vi "Icon_Build 2D Image from Image Cluster.vi"(8 "Error":errorcluster, 11 "Color256":T2={"image type"=0, "image depth"=8, "image"=[210, 210, 210, 210, 210, 210, 210, 210, 210, 210, 210, 210, 210, 210, 210, 210, 210, 210, 210, 210, 210, 210, 210, 210, 210, 210, 210, 210, 210, 210, 210, 210, 210, 210, 210, 210, 210, 210, 5, 5, 5, 210, 210, 5, 5, 210, 210, 210, 5, 5, 5, 210, 210, 5, 210, 210, 210, 5, 210, 210, 210, 210, 210, 210, 210, 210, 210, 210, 210, 210, 210, 5, 210, 210, 5, 210, 210, 5, 210, 5, 210, 210, 210, 5, 210, 5, 5, 210, 210, 5, 210, 210, 210, 210, 210, 210, 210, 210, 210, 210, 210, 210, 210, 5, 210, 210, 5, 210, 210, 210, 210, 5, 210, 210, 210, 5, 210, 5, 210, 5, 210, 5, 210, 210, 210, 210, 210, 210, 210, 210, 210, 210, 210, 210, 210, 5, 210, 210, 5, 210, 210, 5, 210, 5, 210, 210, 210, 5, 210, 5, 210, 210, 5, 5, 210, 210, 210, 210, 210, 210, 210, 210, 210, 210, 210, 210, 5, 5, 5, 210, 210, 5, 5, 210, 210, 210, 5, 5, 5, 210, 210, 5, 210, 210, 210, 5, 210, 210, 210, 210, 210, 210, 210, 210, 210, 210, 210, 210, 210, 210, 210, 210, 210, 210, 210, 210, 210, 210, 210, 210, 210, 210, 210, 210, 210, 210, 210, 210, 210, 210, 210, 210, 210, 210, 210, 5, 5, 5, 5, 5, 5, 5, 5, 5, 5, 5, 5, 5, 5, 5, 5, 5, 5, 5, 5, 5, 5, 5, 5, 5, 5, 5, 5, 5, 5, 210, 210, 5, 5, 5, 5, 5, 5, 5, 5, 5, 5, 5, 5, 5, 5, 5, 5, 5, 5, 5, 5, 5, 5, 5, 5, 5, 5, 5, 5, 5, 5, 210, 210, 5, 5, 5, 5, 5, 5, 5, 5, 5, 5, 5, 5, 5, 5, 5, 5, 5, 5, 5, 5, 5, 5, 5, 5, 5, 5, 5, 5, 5, 5, 210, 210, 5, 5, 210, 210, 5, 5, 210, 210, 210, 5, 5, 210, 210, 210, 210, 5, 5, 210, 210, 5, 5, 210, 210, 210, 5, 210, 210, 210, 210, 5, 210, 210, 5, 210, 5, 5, 210, 5, 210, 5, 5, 210, 5, 210, 5, 5, 5, 5, 210, 5, 5, 210, 5, 5, 210, 5, 5, 210, 5, 5, 5, 5, 210, 210, 5, 210, 5, 5, 5, 5, 210, 210, 210, 5, 5, 210, 210, 210, 5, 5, 210, 210, 210, 210, 5, 5, 210, 5, 5, 210, 210, 210, 5, 5, 210, 210, 5, 210, 5, 5, 210, 5, 210, 5, 5, 210, 5, 210, 5, 5, 5, 5, 210, 5, 5, 210, 5, 5, 210, 5, 5, 210, 5, 5, 5, 5, 210, 210, 5, 5, 210, 210, 5, 5, 210, 5, 5, 210, 5, 210, 210, 210, 210, 5, 210, 5, 5, 210, 5, 5, 210, 5, 5, 210, 210, 210, 210, 5, 210, 210, 5, 5, 5, 5, 5, 5, 5, 5, 5, 5, 5, 5, 5, 5, 5, 5, 5, 5, 5, 5, 5, 5, 5, 5, 5, 5, 5, 5, 5, 5, 210, 210, 5, 5, 5, 5, 5, 5, 5, 5, 5, 5, 5, 5, 5, 5, 5, 5, 5, 5, 5, 5, 5, 5, 5, 5, 5, 5, 5, 5, 5, 5, 210, 210, 5, 5, 5, 5, 5, 5, 5, 5, 5, 5, 5, 210, 210, 210, 5, 5, 210, 210, 210, 5, 5, 5, 5, 5, 5, 5, 5, 5, 5, 5, 210, 210, 5, 5, 5, 5, 5, 5, 5, 5, 5, 5, 5, 5, 5, 5, 210, 5, 210, 5, 5, 210, 5, 5, 5, 5, 5, 5, 5, 5, 5, 5, 210, 210, 5, 5, 5, 5, 5, 5, 5, 5, 5, 5, 5, 5, 210, 210, 5, 5, 210, 5, 5, 210, 5, 5, 5, 5, 5, 5, 5, 5, 5, 5, 210, 210, 5, 5, 5, 5, 5, 5, 5, 5, 5, 5, 5, 210, 5, 5, 5, 5, 210, 5, 5, 210, 5, 5, 5, 5, 5, 5, 5, 5, 5, 5, 210, 210, 5, 5, 5, 5, 5, 5, 5, 5, 5, 5, 5, 210, 210, 210, 210, 5, 210, 210, 210, 5, 5, 5, 5, 5, 5, 5, 5, 5, 5, 5, 210, 210, 5, 5, 5, 5, 5, 5, 5, 5, 5, 5, 5, 5, 5, 5, 5, 5, 5, 5, 5, 5, 5, 5, 5, 5, 5, 5, 5, 5, 5, 5, 210, 210, 5, 5, 5, 5, 5, 5, 5, 5, 5, 5, 5, 5, 5, 5, 5, 5, 5, 5, 5, 5, 5, 5, 5, 5, 5, 5, 5, 5, 5, 5, 210, 210, 5, 5, 5, 5, 210, 210, 5, 5, 210, 210, 210, 5, 5, 210, 210, 210, 5, 5, 5, 210, 210, 5, 5, 210, 5, 5, 5, 210, 5, 5, 210, 210, 5, 5, 5, 210, 5, 5, 210, 5, 210, 5, 5, 210, 5, 210, 5, 5, 210, 5, 210, 5, 5, 210, 5, 5, 210, 5, 210, 5, 5, 5, 210, 210, 5, 5, 5, 210, 210, 210, 210, 5, 210, 210, 210, 5, 5, 210, 210, 210, 5, 5, 210, 210, 210, 210, 5, 5, 5, 210, 5, 5, 5, 5, 210, 210, 5, 5, 5, 210, 5, 5, 210, 5, 210, 5, 5, 210, 5, 210, 5, 5, 210, 5, 210, 5, 5, 210, 5, 5, 5, 210, 5, 5, 5, 5, 210, 210, 5, 5, 5, 210, 5, 5, 210, 5, 210, 5, 5, 210, 5, 210, 5, 5, 210, 5, 210, 5, 5, 210, 5, 5, 5, 210, 5, 5, 5, 5, 210, 210, 5, 5, 5, 5, 5, 5, 5, 5, 5, 5, 5, 5, 5, 5, 5, 5, 5, 5, 5, 5, 5, 5, 5, 5, 5, 5, 5, 5, 5, 5, 210, 210, 5, 5, 5, 5, 5, 5, 5, 5, 5, 5, 5, 5, 5, 5, 5, 5, 5, 5, 5, 5, 5, 5, 5, 5, 5, 5, 5, 5, 5, 5, 210, 210, 210, 210, 210, 210, 210, 210, 210, 210, 210, 210, 210, 210, 210, 210, 210, 210, 210, 210, 210, 210, 210, 210, 210, 210, 210, 210, 210, 210, 210, 210, 210], "mask"=[255, 255, 255, 255, 255, 255, 255, 255, 255, 255, 255, 255, 255, 255, 255, 255, 255, 255, 255, 255, 255, 255, 255, 255, 255, 255, 255, 255, 255, 255, 255, 255, 255, 255, 255, 255, 255, 255, 255, 255, 255, 255, 255, 255, 255, 255, 255, 255, 255, 255, 255, 255, 255, 255, 255, 255, 255, 255, 255, 255, 255, 255, 255, 255, 255, 255, 255, 255, 255, 255, 255, 255, 255, 255, 255, 255, 255, 255, 255, 255, 255, 255, 255, 255, 255, 255, 255, 255, 255, 255, 255, 255, 255, 255, 255, 255, 255, 255, 255, 255, 255, 255, 255, 255, 255, 255, 255, 255, 255, 255, 255, 255, 255, 255, 255, 255, 255, 255, 255, 255, 255, 255, 255, 255, 255, 255, 255, 255], "colors"=[16777215, 16777164, 16777113, 16777062, 16777011, 16776960, 16764159, 16764108, 16764057, 16764006, 16763955, 16763904, 16751103, 16751052, 16751001, 16750950, 16750899, 16750848, 16738047, 16737996, 16737945, 16737894, 16737843, 16737792, 16724991, 16724940, 16724889, 16724838, 16724787, 16724736, 16711935, 16711884, 16711833, 16711782, 16711731, 16711680, 13434879, 13434828, 13434777, 13434726, 13434675, 13434624, 13421823, 13421772, 13421721, 13421670, 13421619, 13421568, 13408767, 13408716, 13408665, 13408614, 13408563, 13408512, 13395711, 13395660, 13395609, 13395558, 13395507, 13395456, 13382655, 13382604, 13382553, 13382502, 13382451, 13382400, 13369599, 13369548, 13369497, 13369446, 13369395, 13369344, 10092543, 10092492, 10092441, 10092390, 10092339, 10092288, 10079487, 10079436, 10079385, 10079334, 10079283, 10079232, 10066431, 10066380, 10066329, 10066278, 10066227, 10066176, 10053375, 10053324, 10053273, 10053222, 10053171, 10053120, 10040319, 10040268, 10040217, 10040166, 10040115, 10040064, 10027263, 10027212, 10027161, 10027110, 10027059, 10027008, 6750207, 6750156, 6750105, 6750054, 6750003, 6749952, 6737151, 6737100, 6737049, 6736998, 6736947, 6736896, 6724095, 6724044, 6723993, 6723942, 6723891, 6723840, 6711039, 6710988, 6710937, 6710886, 6710835, 6710784, 6697983, 6697932, 6697881, 6697830, 6697779, 6697728, 6684927, 6684876, 6684825, 6684774, 6684723, 6684672, 3407871, 3407820, 3407769, 3407718, 3407667, 3407616, 3394815, 3394764, 3394713, 3394662, 3394611, 3394560, 3381759, 3381708, 3381657, 3381606, 3381555, 3381504, 3368703, 3368652, 3368601, 3368550, 3368499, 3368448, 3355647, 3355596, 3355545, 3355494, 3355443, 3355392, 3342591, 3342540, 3342489, 3342438, 3342387, 3342336, 65535, 65484, 65433, 65382, 65331, 65280, 52479, 52428, 52377, 52326, 52275, 52224, 39423, 39372, 39321, 39270, 39219, 39168, 26367, 26316, 26265, 26214, 26163, 26112, 13311, 13260, 13209, 13158, 13107, 13056, 255, 204, 153, 102, 51, 15597568, 14483456, 12255232, 11141120, 8912896, 7798784, 5570560, 4456448, 2228224, 1114112, 60928, 56576, 47872, 43520, 34816, 30464, 21760, 17408, 8704, 4352, 238, 221, 187, 170, 136, 119, 85, 68, 34, 17, 15658734, 14540253, 12303291, 11184810, 8947848, 7829367, 5592405, 4473924, 2236962, 1118481, 0], "Rectangle"={"left"=0, "top"=0, "right"=32, "bottom"=32}}) -> (0 "Error Out":errorcluster, 3 "2D Image Out":T1)   [LabVIEW 2009]
uses:
  Controls/Cluster/Cluster_Image Data.ctl
  Controls/Cluster/CLuster_Selectoin Box.ctl
  Controls/Array/Color Box Array_2D Icon Viewer.ctl
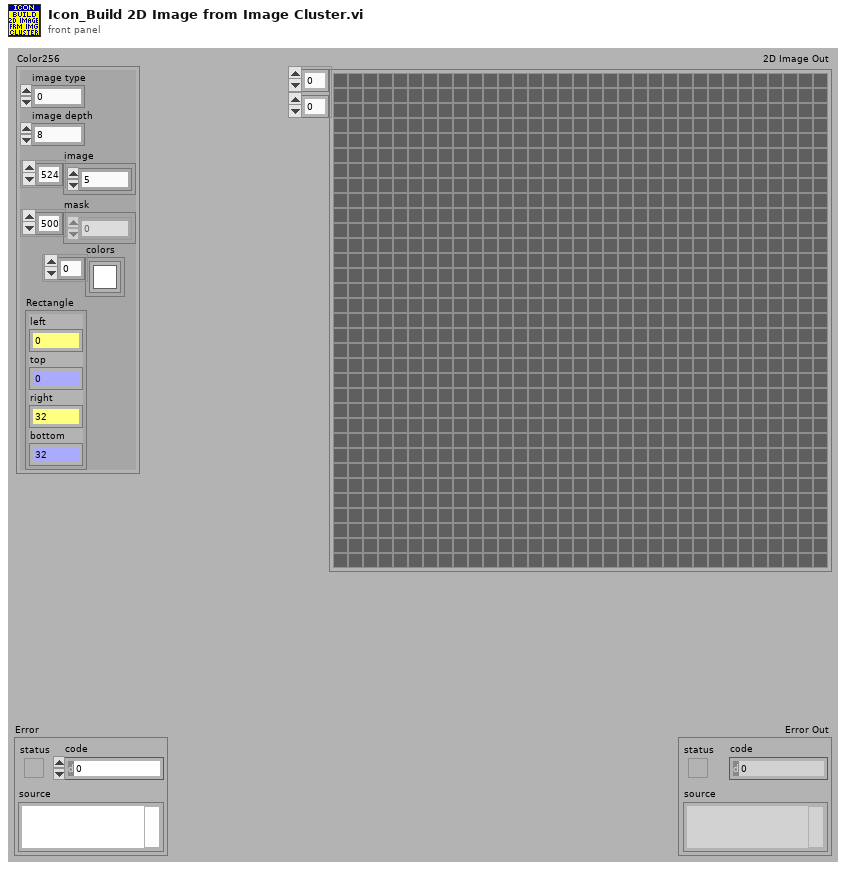
[diagram p1: front panel]
types:
  T1 = typedef "Color Box Array_2D Icon Viewer.ctl" = u32[][]
  T2 = typedef "Cluster_Image Data.ctl" = cluster{"image type":i32, "image depth":i32, "image":u8[], "mask":u8[], "colors":u32[], "Rectangle":T3}
  T3 = typedef "CLuster_Selectoin Box.ctl" = cluster{"left":i16, "top":i16, "right":i16, "bottom":i16}
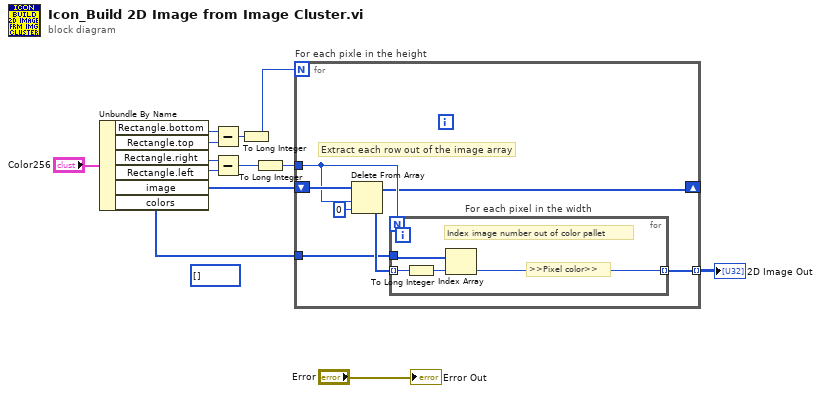
[diagram p0: block diagram]
diagram:
  (unwired) u32[] [] ("colors")
  n1 = Unbundle By Name("Color256") -> ("Rectangle.bottom"=w6:i16, "Rectangle.top"=w5:i16, "Rectangle.right"=w13:i16, "Rectangle.left"=w12:i16, "image"=w9:u8[], "colors"=w8:u32[])
  n2 = Subtract(x=w6, y=w5) -> (x-y=w11:i16)
  n3 = Subtract(x=w13, y=w12) -> (x-y=w10:i16)
  n4 = To Long Integer(number=w11) -> (32bit integer=w1:i32)
  n5 = To Long Integer(number=w10) -> (32bit integer=w2:i32)
  n6 = for "For each pixle in the height" {
    N: w1 -> [_]
    tunnel: w2 -> [w18]
    shift-right: [w16] -> _
    shift-left: w9 -> [w20]
    tunnel: w8 -> [w15]
    tunnel: [w14] -> w4 mode=indexing
    # "Extract each row out of the image array"
    n7 = Delete From Array(array=w20, length=w18, index=0) -> (deleted portion=w17:u8[], array with subset deleted=w16:u8[])
    n8 = for "For each pixel in the width" {
      N: w18 -> [_]
      tunnel: w17 -> [w23] mode=indexing
      tunnel: w15 -> [w24]
      tunnel: [w22] -> w14 mode=indexing
      # ">>Pixel color>>"
      # "Index image number out of color pallet"
      n9 = To Long Integer(number=w23) -> (32bit integer=w21:i32)
      n10 = Index Array(array=w24, index=w21) -> (element=w22:u32)
    }
  }
  "2D Image Out" <- w4
  "Error Out" <- "Error"
